vi "GetLoopTime.vi"(6 "Legacy (f)?":bool, 8 "error in (no error)":errorcluster) -> (0 "error out":errorcluster, 2 "LoopTime":u32)   [LabVIEW 2011]
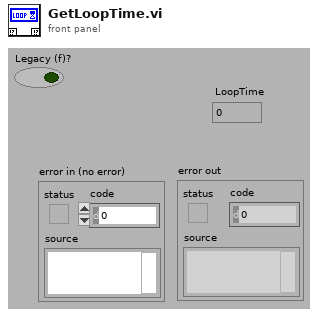
[diagram p1: front panel]
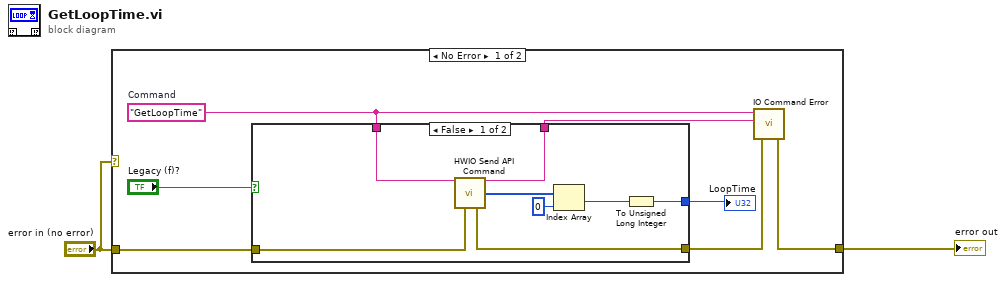
[diagram p0: block diagram]
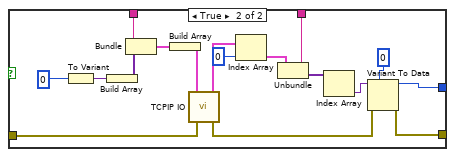
[diagram p2: hidden frame]
diagram:
  n1 = case shown="No Error" "error in (no error)" {
    tunnel: "error in (no error)" -> [w8 w35]
    tunnel: [w6 w35] -> w2
    frame No Error {
      w5 = "GetLoopTime"  # Command
      n2 = case shown="False" "Legacy (f)?" {
        tunnel: [w11 w29] -> w9
        tunnel: w8 -> [w17 w27]
        tunnel: [w16 w26] -> w7
        tunnel: w5 -> [w14 w25]
        tunnel: [w15 w24] -> w4
        frame False {
          n3 = call "HWIO Send API Command.vi"("Action"=w14, "error in (no error)"=w17) -> ("Action out"=w15:string, "Integer out"=w13:i32[], "error out"=w16:errorcluster)  [unwired: 6 in, 5 out]
          n4 = Index Array(array=w13, index=0) -> (element=w10:i32)
          n5 = To Unsigned Long Integer(number=w10) -> (unsigned 32bit integer=w11:u32)
        }
        frame True {
          n6 = To Variant(anything=u32 0) -> (Variant=w34:variant)
          n7 = Build Array(w34) -> (w32:variant[])
          n8 = Bundle("Command"=w25, w32) -> (w31:cluster{"Command":string, variant[]})  [unwired: 1 out]
          n9 = Build Array(w31) -> (w22:cluster{"Command":string, variant[]}[])
          n10 = call "TCPIP IO.vi"("error in (no error)"=w27, "Commands"=w22) -> ("error out"=w28:errorcluster, "Responses"=w23:cluster{string, variant[]}[])  [unwired: 1 in, 3 out]
          n11 = Index Array(array=w23, index=0) -> (element=w21:cluster{string, variant[]})
          n12 = Unbundle(w21) -> (w24:string, w19:variant[])
          n13 = Index Array(array=w19) -> (element=w20:variant)  [unwired: 1 in]
          n14 = Variant To Data(error in=w28, type=u32 0, Variant=w20) -> (data=w29:u32, error out=w26:errorcluster)
        }
      }
      "LoopTime" <- w9
      n15 = call "IO Command Error.vi"("error in (no error)"=w7, "Command Returned (\"\")"=w4, "Command Sent (\"\")"=w5) -> ("error out"=w6:errorcluster)  [unwired: 4 out]
    }
    frame Error {
    }
  }
  "error out" <- w2
